vi "Local_Sense_Test_v1.vi"(10 "HMP VISA":refnum<visa-resource-name>, 11 "Control Board VISA":refnum<visa-resource-name>) -> (3 "Pass?":bool)   [LabVIEW 2019]
uses:
  Ctls/Powersupply_Auto_Enum_v1.ctl
panel:
  out "MSE Array":dbl[](array[numeric])
  out "Voltage Readings":dbl[][](array[numeric])
  out "Message OUT":string
  in  "Message IN":string
  out "error out":errorcluster
  in  "error in (no error)":errorcluster
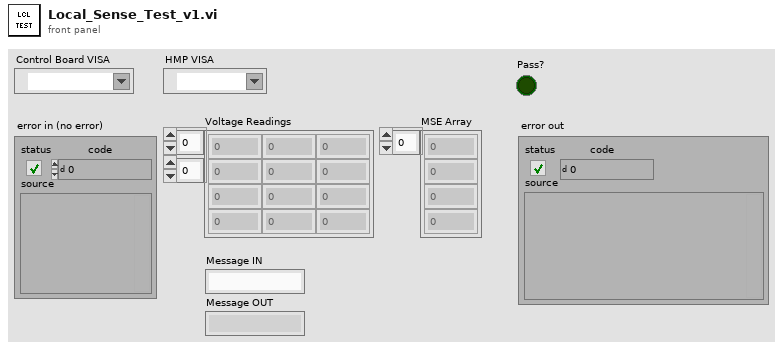
[diagram p1: front panel]
types:
  T1 = typedef "Powersupply_Auto_Enum_v1.ctl" = enum16{"Off", "Control Power", "HMP2020 Control + DC32V", "HMP2020 Control + DC8V", "HMP4040 Control + DC32V", "HMP4040 Control +DC8V"}
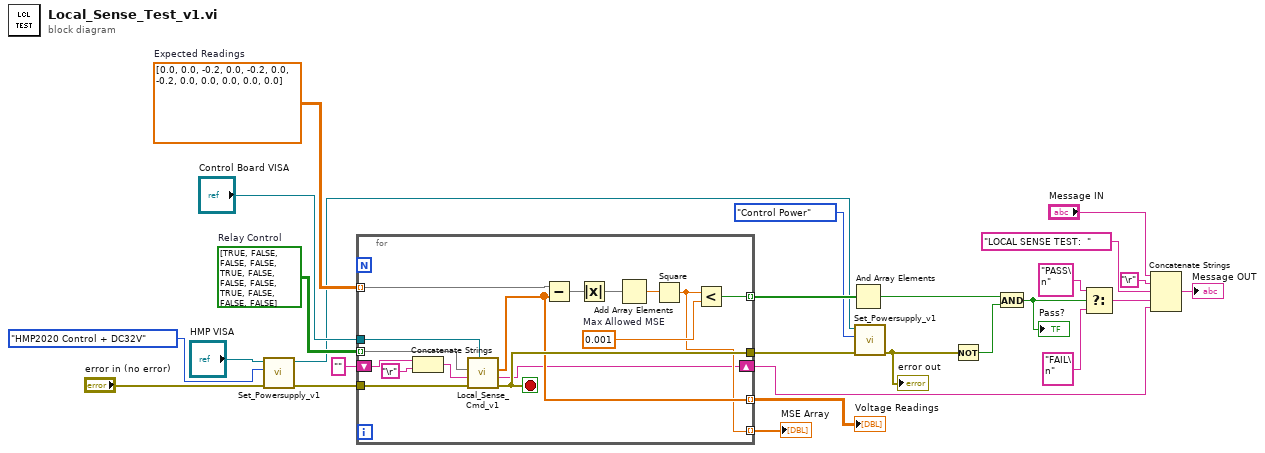
[diagram p0: block diagram]
diagram:
  w9 = dbl[][] [[0.0, 0.0, -0.2], [0.0, -0.2, 0.0], [-0.2, 0.0, 0.0], [0.0, 0.0, 0.0]]  # Expected Readings
  w25 = bool[][] [[TRUE, FALSE, FALSE], [FALSE, TRUE, FALSE], [FALSE, FALSE, TRUE], [FALSE, FALSE, FALSE]]  # Relay Control
  n1 = call "Set_Powersupply_v1.vi"("error in (no error)"="error in (no error)", "Enum"=Powersupply_Auto_Enum_v1."HMP2020 Control + DC32V", "HMP VISA"="HMP VISA") -> ("error out"=w8:errorcluster, "HMP VISA Out"=w2:refnum<visa-resource-name>)  [unwired: 7 in]
  n2 = for {
    tunnel: [w41] -> w4
    tunnel: w8 -> [w42]
    tunnel: w9 -> [w38] mode=indexing
    tunnel: [w35] -> w26 mode=indexing
    tunnel: w25 -> [w34] mode=indexing
    tunnel: [w33] -> w22 mode=indexing
    tunnel: [w32] -> w21 mode=indexing
    shift-right: [w31] -> w14
    shift-left: "" -> [w30]
    tunnel: "Control Board VISA" -> [w27]
    stop <- w41 stop-if-true
    w36 = 0.001  # Max Allowed MSE
    n3 = Concatenate Strings(w30, "\r") -> (w29:string)
    n4 = call "Local_Sense_Cmd_v1.vi"("Control Board VISA"=w27, "error in (no error)"=w42, "Message IN"=w29, "Relay Control"=w34) -> ("error out"=w41:errorcluster, "Message OUT"=w31:string, "Voltage Array"=w33:dbl[])  [unwired: 4 in, 1 out]
    n5 = Subtract(x=w38, y=w33) -> (x-y=w40:dbl[])
    n6 = Absolute Value(x=w40) -> (abs(x)=w39:dbl[])
    n7 = Add Array Elements(numeric array=w39) -> (sum=w37:dbl)
    n8 = Square(x=w37) -> (x^2=w32:dbl)
    n9 = Less?(x=w32, y=w36) -> (x < y?=w35:bool)
  }
  "Voltage Readings" <- w22
  "MSE Array" <- w21
  n10 = And Array Elements(Boolean array=w26) -> (logical AND=w24:bool)
  n11 = call "Set_Powersupply_v1.vi"("error in (no error)"=w4, "Enum"=Powersupply_Auto_Enum_v1."Control Power", "HMP VISA"=w2) -> ("error out"=w3:errorcluster)  [unwired: 7 in, 1 out]
  "error out" <- w3
  n12 = Not(x=w3) -> (.not. x?=w23:bool)
  n13 = And(x=w24, y=w23) -> (x .and. y?=w16:bool)
  "Pass?" <- w16
  n14 = Select(t="PASS\n", s=w16, f="FAIL\n") -> (s? t:f=w15:string)
  n15 = Concatenate Strings("Message IN", "\r", "LOCAL SENSE TEST:  ", w15, w14) -> (→"Message OUT":string)
